vi "pointToSegmnetDistPastT.vi"(10 "point":cluster{"X":sgl, "Y":sgl}, 11 "Line Segment":T1) -> (0 "t":dbl, 1 "onSegment":bool, 3 "distance":dbl, 4 "y-dist":dbl, 6 "x-Dist":dbl)   [LabVIEW 2015]
uses:
  <vilib>/Analysis/baseanly.llb/Real Dot Product.vi
  <vilib>/Analysis/NI_AALBase.lvlib
panel:
  out "lineDistance":sgl
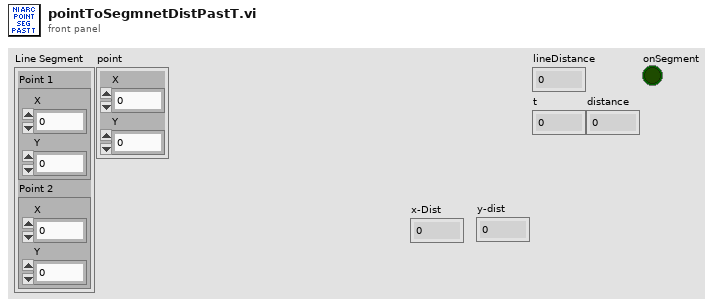
[diagram p1: front panel]
types:
  T1 = cluster{"Point 1":cluster{"X":sgl, "Y":sgl}, "Point 2":cluster{"X":sgl, "Y":sgl}}
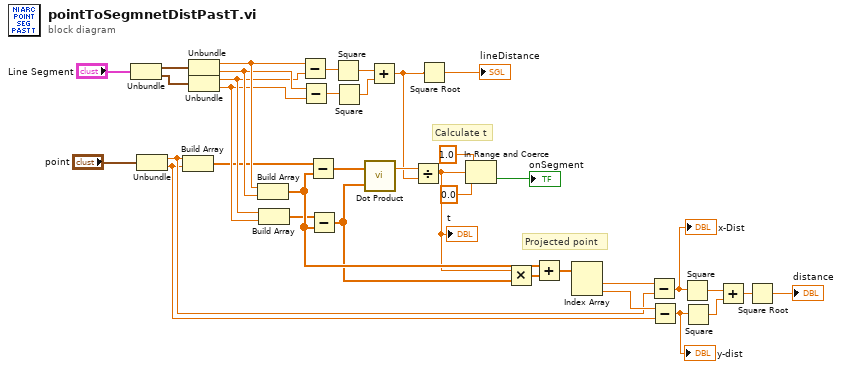
[diagram p0: block diagram]
diagram:
  # "Projected point"
  # "Calculate t"
  n1 = Unbundle("Line Segment") -> ("Point 1"=w35:cluster{"X":sgl, "Y":sgl}, "Point 2"=w34:cluster{"X":sgl, "Y":sgl})
  n2 = Unbundle("point") -> ("X"=w9:sgl, "Y"=w8:sgl)
  n3 = Build Array(w9, w8) -> (w24:sgl[])
  n4 = Unbundle(w35) -> ("X"=w28:sgl, "Y"=w27:sgl)
  n5 = Unbundle(w34) -> ("X"=w26:sgl, "Y"=w25:sgl)
  n6 = Build Array(w28, w27) -> (w19:sgl[])
  n7 = Build Array(w26, w25) -> (w18:sgl[])
  n8 = Subtract(x=w28, y=w26) -> (x-y=w33:sgl)
  n9 = Subtract(x=w27, y=w25) -> (x-y=w32:sgl)
  n10 = Subtract(x=w24, y=w19) -> (x-y=w23:sgl[])
  n11 = Subtract(x=w18, y=w19) -> (x-y=w16:sgl[])
  n12 = Square(x=w33) -> (x^2=w31:sgl)
  n13 = Square(x=w32) -> (x^2=w30:sgl)
  n14 = call-poly <vilib>:"Dot Product.vi"("Y Vector"=w16, "X Vector"=w23) -> ("X * Y"=w22:dbl)  [unwired: 1 out]
  n15 = Add(x=w31, y=w30) -> (x+y=w3:sgl)
  n16 = Divide(x=w22, y=w3) -> (x/y=w1:dbl)
  "t" <- w1
  n17 = Square Root(x=w3) -> (sqrt(x)=→"lineDistance":sgl)
  n18 = In Range and Coerce(upper limit=1.0, x=w1, lower limit=0.0) -> (In Range?=→"onSegment":bool)  [unwired: 1 out]
  n19 = Multiply(x=w1, y=w16) -> (x*y=w17:dbl[])
  n20 = Add(x=w19, y=w17) -> (x+y=w15:dbl[])
  n21 = Index Array(array=w15) -> (element #1=w11:dbl, element #2=w10:dbl)  [unwired: 2 in]
  n22 = Subtract(x=w11, y=w9) -> (x-y=w12:dbl)
  "x-Dist" <- w12
  n23 = Subtract(x=w10, y=w8) -> (x-y=w4:dbl)
  "y-dist" <- w4
  n24 = Square(x=w12) -> (x^2=w13:dbl)
  n25 = Square(x=w4) -> (x^2=w14:dbl)
  n26 = Add(x=w13, y=w14) -> (x+y=w7:dbl)
  n27 = Square Root(x=w7) -> (sqrt(x)=→"distance":dbl)
